vi "Release.vi"(8 "error in (no error)":errorcluster, 11 "StepperMotor in":refnum<class "StepperMotor.lvclass">) -> (0 "error out":errorcluster, 3 "StepperMotor out":refnum<class "StepperMotor.lvclass">)   [LabVIEW 2022 SP3, in "Motorshield.lvlib" / "StepperMotor.lvclass"]
uses:
  StepperMotor.lvclass
  StepperMotor.lvclass/StepperMotor.ctl
  Motorshield/Motorshield.lvclass
  C:/Users/Carlos/Desktop/onlab/source/Motorshield/Motorshield/Motorshield.lvclass
  C:/Users/Carlos/Desktop/onlab/source/Motorshield/StepperMotor/StepperMotor.lvclass
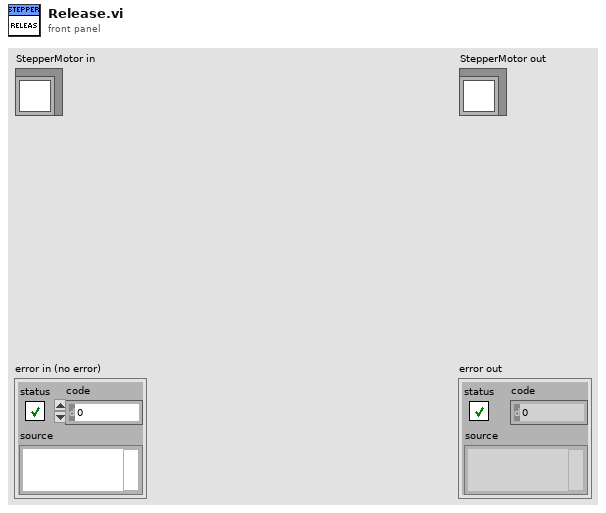
[diagram p1: front panel]
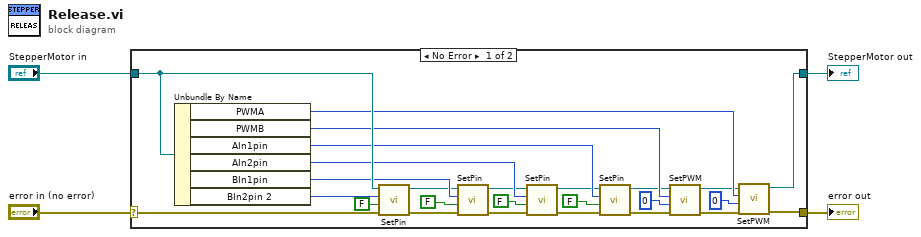
[diagram p0: block diagram]
diagram:
  n1 = case shown="No Error" "error in (no error)" {
    selector: "error in (no error)" -> [w30 w32]
    tunnel: [w7 w32] -> w3
    tunnel: [w9 w31] -> w1
    tunnel: "StepperMotor in" -> [w28 w31]
    frame No Error {
      n2 = Unbundle By Name(w28) -> ("PWMA"=w12:u8, "PWMB"=w13:u8, "AIn1pin"=w23:u8, "AIn2pin"=w26:u8, "BIn1pin"=w27:u8, "BIn2pin 2"=w29:u8)
      n3 = call "SetPin.vi"("error in (no error)"=w30, "Value"=FALSE, "Led num"=w29, "Motorshield in"=w28) -> ("error out"=w21:errorcluster, "Motorshield out"=w25:refnum<class "StepperMotor.lvclass">)  [unwired: 6 in]
      n4 = call "SetPin.vi"("error in (no error)"=w21, "Value"=FALSE, "Led num"=w27, "Motorshield in"=w25) -> ("error out"=w20:errorcluster, "Motorshield out"=w24:refnum<class "StepperMotor.lvclass">)  [unwired: 6 in]
      n5 = call "SetPin.vi"("error in (no error)"=w20, "Value"=FALSE, "Led num"=w26, "Motorshield in"=w24) -> ("error out"=w19:errorcluster, "Motorshield out"=w22:refnum<class "StepperMotor.lvclass">)  [unwired: 6 in]
      n6 = call "SetPin.vi"("error in (no error)"=w19, "Value"=FALSE, "Led num"=w23, "Motorshield in"=w22) -> ("error out"=w14:errorcluster, "Motorshield out"=w11:refnum<class "StepperMotor.lvclass">)  [unwired: 6 in]
      n7 = call "SetPWM.vi"("error in (no error)"=w14, "Value"=u16 0, "Led num"=w13, "Motorshield in"=w11) -> ("error out"=w8:errorcluster, "Motorshield out"=w10:refnum<class "StepperMotor.lvclass">)  [unwired: 6 in]
      n8 = call "SetPWM.vi"("error in (no error)"=w8, "Value"=u16 0, "Led num"=w12, "Motorshield in"=w10) -> ("error out"=w7:errorcluster, "Motorshield out"=w9:refnum<class "StepperMotor.lvclass">)  [unwired: 6 in]
    }
    frame Error {
    }
  }
  "error out" <- w3
  "StepperMotor out" <- w1
